vi "3D Display.vi"(8 "Yaw":dbl(knob) scale=0.0..360.0, 9 "Roll":dbl(knob) scale=0.0..360.0, 10 "Pitch":dbl(knob) scale=0.0..360.0, 11 "Object Refnum In":refnum<vi>) -> (3 "Object Refnum Out":refnum<vi>)   [LabVIEW 2015]
uses:
  <vilib>/picture/3D Picture Control/NI_3D Picture Control.lvlib
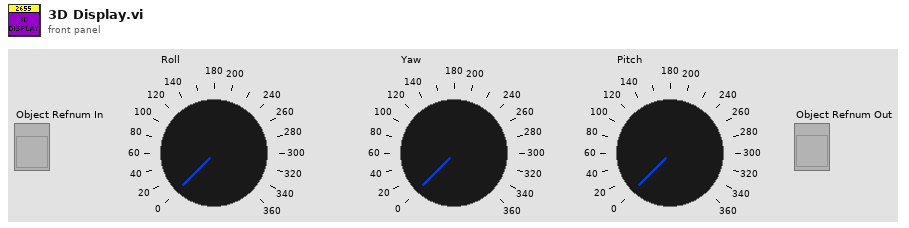
[diagram p1: front panel]
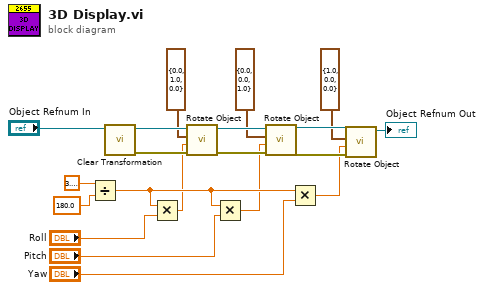
[diagram p0: block diagram]
diagram:
  n1 = Divide(x=3.141592653589793, y=180.0) -> (x/y=w10:dbl)
  n2 = call <vilib>:"Clear Transformation.vi"("Object Refnum In"="Object Refnum In") -> ("error out"=w17:errorcluster, "Object Refnum Out"=w18:refnum<vi>)  [unwired: 9 in]
  n3 = Multiply(x=w10, y="Roll") -> (x*y=w8:dbl)
  n4 = call <vilib>:"Rotate Object.vi"("error in (no error)"=w17, "Angle"=w8, "Axis"=cluster{"X":sgl, "Y":sgl, "Z":sgl} {"X"=0.0, "Y"=1.0, "Z"=0.0}, "Scene.Object In"=w18) -> ("error out"=w19:errorcluster, "Scene.Object Out"=w20:refnum<vi>)  [unwired: 6 in]
  n5 = Multiply(x=w10, y="Pitch") -> (x*y=w7:dbl)
  n6 = call <vilib>:"Rotate Object.vi"("error in (no error)"=w19, "Angle"=w7, "Axis"=cluster{"X":sgl, "Y":sgl, "Z":sgl} {"X"=0.0, "Y"=0.0, "Z"=1.0}, "Scene.Object In"=w20) -> ("error out"=w13:errorcluster, "Scene.Object Out"=w14:refnum<vi>)  [unwired: 6 in]
  n7 = Multiply(x=w10, y="Yaw") -> (x*y=w9:dbl)
  n8 = call <vilib>:"Rotate Object.vi"("error in (no error)"=w13, "Angle"=w9, "Axis"=cluster{"X":sgl, "Y":sgl, "Z":sgl} {"X"=1.0, "Y"=0.0, "Z"=0.0}, "Scene.Object In"=w14) -> ("Scene.Object Out"=→"Object Refnum Out":refnum<vi>)  [unwired: 6 in, 1 out]
